vi "timing.vi"() -> ()   [LabVIEW 2019]
panel:
  out "end time":string
  out "start time":string
  out "time elapsed":dbl format="%.2f"
  out "time string":string
  out "Exposure":dbl(slide)=84.475 scale=0.0..0.2 scale format="%.1f"
  in  "StdBy":string="Standing By"
  in  "Standby?":bool
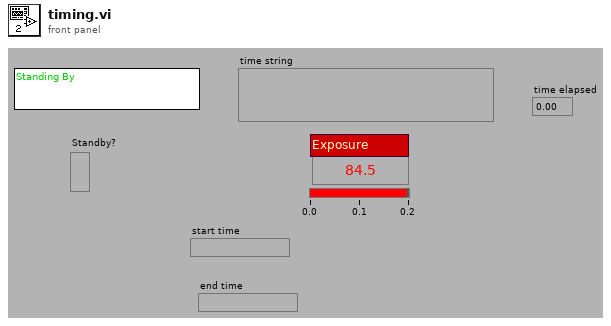
[diagram p1: front panel]
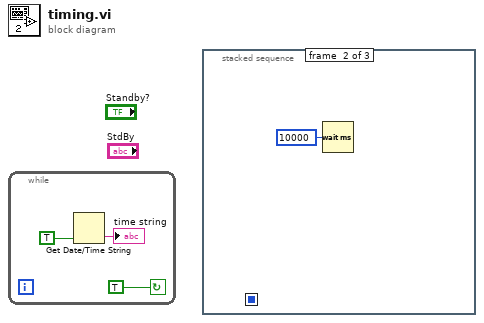
[diagram p0: block diagram]
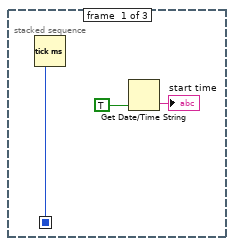
[diagram p2: hidden frame]
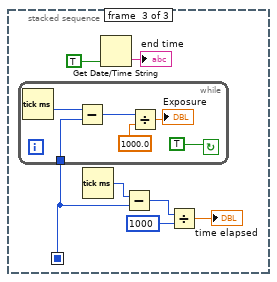
[diagram p3: hidden frame]
diagram:
  n1 = while {
    stop <- TRUE continue-if-true
    n2 = Get Date/Time String(want seconds? (F)=TRUE) -> (time string=→"time string":string)  [unwired: 2 in, 1 out]
  }
  n3 = stacked-sequence {
    seq-local: [w6 _ _] -> [_ _ w12]
    frame #0 {
      n4 = Tick Count (ms)() -> (millisecond timer value=w6:u32)
      n5 = Get Date/Time String(want seconds? (F)=TRUE) -> (time string=→"start time":string)  [unwired: 2 in, 1 out]
    }
    frame #1 {
      n6 = Wait (ms)(milliseconds to wait=u32 10000 ("millisecond multiple")) -> ()  [unwired: 1 out]
    }
    frame #2 {
      n7 = while {
        tunnel: w12 -> [w16]
        stop <- TRUE continue-if-true
        n8 = Tick Count (ms)() -> (millisecond timer value=w18:u32)
        n9 = Subtract(x=w18, y=w16) -> (x-y=w17:u32)
        n10 = Divide(x=w17, y=1000.0) -> (x/y=→"Exposure":dbl)
      }
      n11 = Tick Count (ms)() -> (millisecond timer value=w13:u32)
      n12 = Get Date/Time String(want seconds? (F)=TRUE) -> (time string=→"end time":string)  [unwired: 2 in, 1 out]
      n13 = Subtract(x=w13, y=w12) -> (x-y=w11:u32)
      n14 = Divide(x=w11, y=u32 1000) -> (x/y=→"time elapsed":dbl)
    }
  }
